vi "InterceptPassTactic_v2_Init.vi"(0 "object in":refnum<class "InterceptPassTactic_v2.lvclass">, 5 "error in (no error)":errorcluster) -> (14 "object out":refnum<class "InterceptPassTactic_v2.lvclass">, 19 "error out":errorcluster)   [LabVIEW 2023, in "InterceptPassTactic_v2.lvclass"]
uses:
  InterceptPassTactic_v2.lvclass
  C:/Users/ebert/Documents/codes/SSL/repo/SSL_AI/NewSTP/NewTactics/Tactic_v2_class/Tactic_v2.lvclass
  InterceptBallSkill_class/InterceptBallSkill.lvclass
  C:/Users/ebert/Documents/codes/SSL/repo/SSL_AI/NewSTP/NewSkills/Skill_v2_class/Skill_v2.lvclass
  OneTouchPassSkill_class/OneTouchPassSkill.lvclass
  C:/Users/ebert/Documents/codes/SSL/repo/SSL_AI/InterceptBallSkill_class/InterceptBallSkill.lvclass
  OneTouchShotSkill_class/OneTouchShotSkill.lvclass
  NewSTP/NewTactics/Tactic_v2_class/Tactic_v2.lvclass
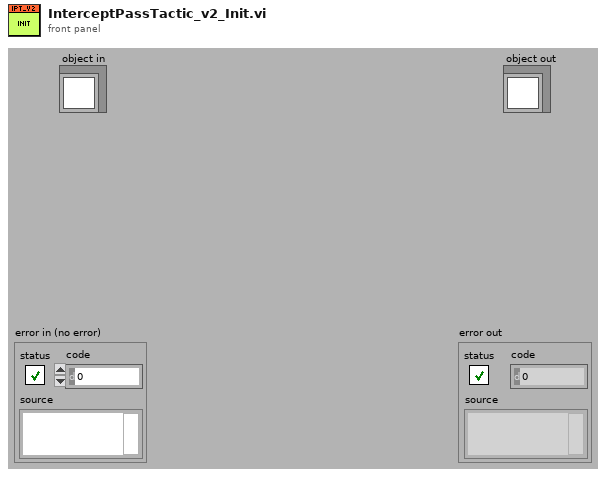
[diagram p1: front panel]
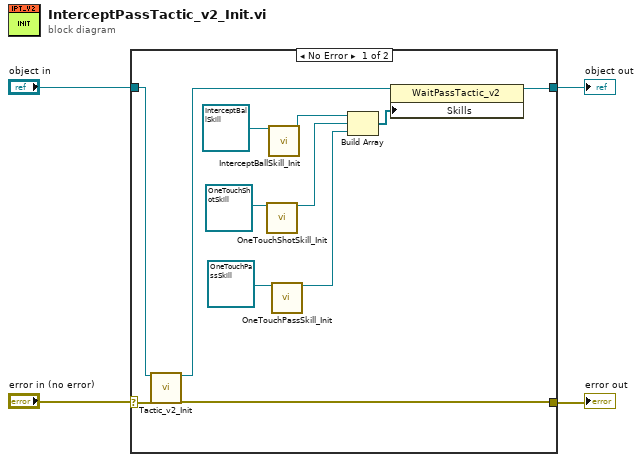
[diagram p0: block diagram]
diagram:
  n1 = case shown="No Error" "error in (no error)" {
    selector: "error in (no error)" -> [w15 w17]
    tunnel: "object in" -> [w16 w18]
    tunnel: [w12 w18] -> w3
    tunnel: [w14 w17] -> w1
    frame No Error {
      n2 = call "Tactic_v2_Init.vi"("object in"=w16, "error in (no error)"=w15) -> ("object out"=w13:refnum<class "InterceptPassTactic_v2.lvclass">, "error out"=w14:errorcluster)  [unwired: 16 in]
      n3 = call "OneTouchShotSkill_Init.vi"("object in"=refnum<class "OneTouchShotSkill.lvclass"> refnum ("OneTouchShotSkill")) -> ("object out"=w8:refnum<class "OneTouchShotSkill.lvclass">)  [unwired: 17 in, 1 out]
      n4 = call "InterceptBallSkill_Init.vi"("object in"=refnum<class "InterceptBallSkill.lvclass"> refnum ("InterceptBallSkill")) -> ("object out"=w5:refnum<class "InterceptBallSkill.lvclass">)  [unwired: 17 in, 1 out]
      n5 = call "OneTouchPassSkill_Init.vi"("object in"=refnum<class "OneTouchPassSkill.lvclass"> refnum ("OneTouchShotSkill")) -> ("object out"=w7:refnum<class "OneTouchPassSkill.lvclass">)  [unwired: 17 in, 1 out]
      n6 = Build Array(w5, w8, w7) -> (w11:refnum<class "InterceptBallSkill.lvclass">[])
      n7 = property class="WaitPassTactic_v2"(reference=w13, "Skills"=w11) -> (reference out=w12:refnum<class "InterceptPassTactic_v2.lvclass">)  [unwired: 1 in, 1 out]
    }
    frame Error {
    }
  }
  "object out" <- w3
  "error out" <- w1
